vi "deeplabV3_preprocess.vi"(8 "error in (no error)":errorcluster, 11 "img":refnum<class "Mat_8U.lvclass">) -> (0 "error out":errorcluster, 3 "blob":refnum<class "Mat_32F.lvclass">)   [LabVIEW 2018]
uses:
  <vilib>/addons/VIRobotics/opencv_yiku/Mat/Mat_8U/Mat_8U.lvclass
  C:/Program Files/National Instruments/LabVIEW 2018_64bit/vi.lib/addons/VIRobotics/opencv_yiku/Mat/Mat/Mat.lvclass
  <vilib>/addons/VIRobotics/opencv_yiku/Mat/Mat_32F/Mat_32F.lvclass
  <vilib>/addons/VIRobotics/opencv_yiku/ctls/scalar3.ctl
  <vilib>/addons/VIRobotics/opencv_yiku/Mat/Create_Mat_32F.vi
  <vilib>/addons/VIRobotics/opencv_yiku/opencv_yiku.lvlib
  <vilib>/addons/VIRobotics/opencv_yiku/Mat/Mat/Mat.lvclass
  <vilib>/addons/VIRobotics/opencv_yiku/Mat/Create_Mat_8U.vi
  <vilib>/addons/VIRobotics/opencv_yiku/Mat/Mat/Mat_release.vi
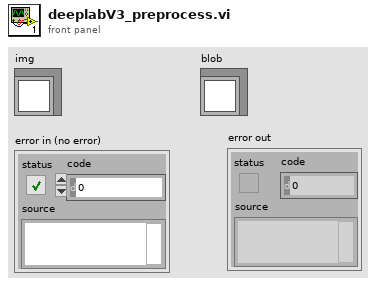
[diagram p1: front panel]
types:
  T1 = typedef "opencv_yiku.lvlib/scalar3.ctl" = cluster{"x":dbl, "y":dbl, "z":dbl}
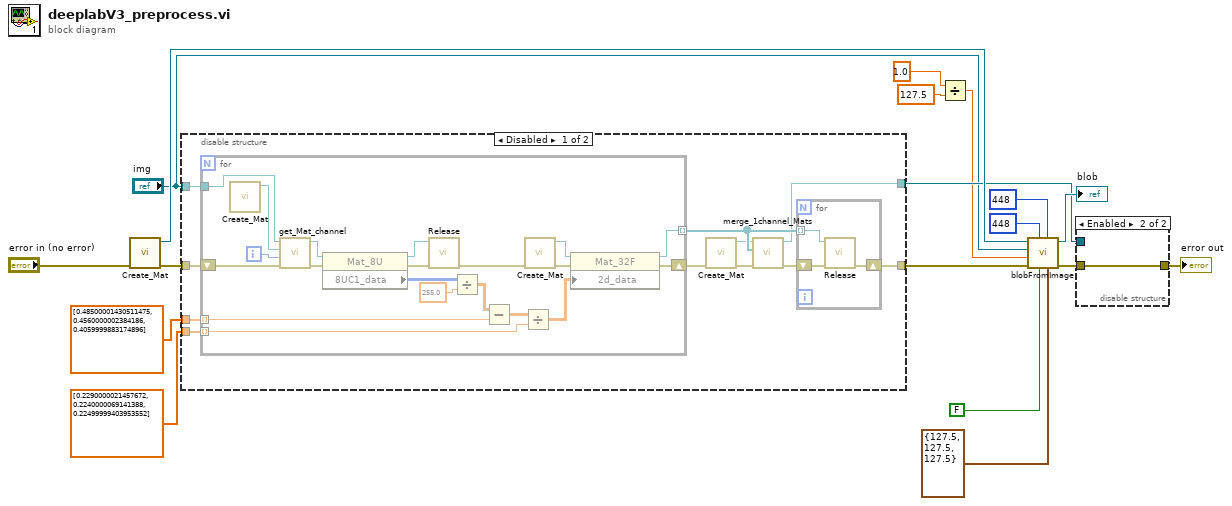
[diagram p0: block diagram]
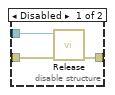
[diagram p2: hidden frame]
diagram:
  n1 = call-poly <vilib>:"Create_Mat.vi"("error in (no error)"="error in (no error)") -> ("error out"=w18:errorcluster, "Mat_32F_out"=w12:refnum<class "Mat_32F.lvclass">)  [unwired: 9 in]
  n2 = disable-structure shown="Disabled" {
    disable-tunnel: w18 -> [w29 w53]
    disable-tunnel: [w28 w53] -> w17
    disable-tunnel: sgl[] [0.229, 0.224, 0.225] -> [w24 _]
    disable-tunnel: sgl[] [0.485, 0.456, 0.406] -> [w23 _]
    disable-tunnel: [w20 _] -> w9
    disable-tunnel: "img" -> [w19 _]
    frame Disabled {
      n3 = for {
        tunnel: w19 -> [w52]
        tunnel: w23 -> [w44] mode=indexing
        tunnel: w24 -> [w42] mode=indexing
        tunnel: [w37] -> w26 mode=indexing
        shift-right: [w35] -> w22
        shift-left: w29 -> [w36]
        i -> [w50]
        n4 = call-poly <vilib>:"Create_Mat.vi"() -> ("Mat_8U_out"=w51:refnum<class "Mat_8U.lvclass">)  [unwired: 10 in, 1 out]
        n5 = call <vilib>:"get_Mat_channel.vi"("error in (no error)"=w36, "channel"=w50, "dst"=w51, "Mat in"=w52) -> ("error out"=w49:errorcluster, "dst out"=w48:refnum<class "Mat_8U.lvclass">)  [unwired: 6 in]
        n6 = property class="Mat_8U"(reference=w48, error in=w49) -> (reference out=w41:refnum<class "Mat_8U.lvclass">, error out=w34:errorcluster, "8UC1_data"=w47:u8[][])
        n7 = call-poly <vilib>:"Release.vi"("error in (no error)"=w34, "Mat in"=w41) -> ("error out"=w40:errorcluster)  [unwired: 9 in]
        n8 = Divide(x=w47, y=sgl 255.0) -> (x/y=w45:sgl[][])
        n9 = Subtract(x=w45, y=w44) -> (x-y=w43:sgl[][])
        n10 = Divide(x=w43, y=w42) -> (x/y=w38:sgl[][])
        n11 = call-poly <vilib>:"Create_Mat.vi"("error in (no error)"=w40) -> ("error out"=w33:errorcluster, "Mat_32F_out"=w39:refnum<class "Mat_32F.lvclass">)  [unwired: 9 in]
        n12 = property class="Mat_32F"(reference=w39, error in=w33, "2d_data"=w38) -> (reference out=w37:refnum<class "Mat_32F.lvclass">, error out=w35:errorcluster)
      }
      n13 = call-poly <vilib>:"Create_Mat.vi"("error in (no error)"=w22) -> ("error out"=w21:errorcluster, "Mat_32F_out"=w25:refnum<class "Mat_32F.lvclass">)  [unwired: 9 in]
      n14 = call <vilib>:"merge_1channel_Mats.vi"("error in (no error)"=w21, "MatArray"=w26, "dst"=w25) -> ("error out"=w27:errorcluster, "dst out"=w20:refnum<class "Mat_32F.lvclass">)  [unwired: 7 in]
      n15 = for {
        tunnel: w26 -> [w32] mode=indexing
        shift-right: [w30] -> w28
        shift-left: w27 -> [w31]
        n16 = call-poly <vilib>:"Release.vi"("error in (no error)"=w31, "Mat in"=w32) -> ("error out"=w30:errorcluster)  [unwired: 9 in]
      }
    }
    frame Enabled {
    }
  }
  n17 = Divide(x=1.0, y=127.5) -> (x/y=w2:dbl)
  n18 = call <vilib>:"blobFromImage.vi"("mean"=T1 {"x"=127.5, "y"=127.5, "z"=127.5}, "rows"=448, "swapRB"=FALSE, "columns"=448, "error in (no error)"=w17, "scale"=w2, "Mat in"="img", "dst"=w12) -> ("error out"=w10:errorcluster, "dst out"=→"blob":refnum<class "Mat_32F.lvclass">)  [unwired: 2 in]
  n19 = disable-structure shown="Enabled" {
    disable-tunnel: w10 -> [w56 w57]
    disable-tunnel: w9 -> [w55 _]
    disable-tunnel: [w54 w57] -> w8
    frame Disabled {
      n20 = call-poly <vilib>:"Release.vi"("error in (no error)"=w56, "Mat in"=w55) -> ("error out"=w54:errorcluster)  [unwired: 9 in]
    }
    frame Enabled {
    }
  }
  "error out" <- w8
